vi "String.Int to String, Small Profile.vi"(11 "Numeric":i32) -> (3 "String":string)   [LabVIEW 2018]
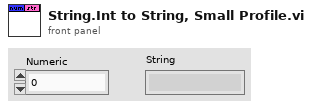
[diagram p1: front panel]
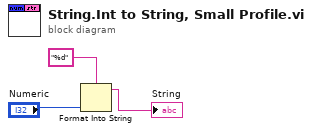
[diagram p0: block diagram]
diagram:
  n1 = Format Into String(format string="%d", "Numeric") -> (resulting string=→"String":string)  [unwired: 2 in, 1 out]
